vi "MassData Parameter Support Demo.vi"() -> ()   [LabVIEW 2017]
uses:
  addons/MassData-Parameter/Utility/Def-MassData Status Indicator(Vertical).ctl
  e399a5d2-a107-417c-bf24-9f3d5e5cdf18.vi
  6831a10e-81b1-43f0-9df7-fec7c9a78c49.vi
  49f32103-30ee-4ef6-a51c-53b3f34b46c3.vi
  addons/MassData-Parameter/_support/FGV-MassData(lvlibp).vi
  <userlib>/_NEVSTOP/Communicable State Machine(CSM)/Utility/CSM Data Type String.vi
  addons/MassData-Parameter/CSM MassData Parameter Support.lvlib
panel:
  in  "Boolean":bool
  in  "stop":bool
  out "MassData Status":T1={"w"={287840.0, 276144.0}, "r"={287840.0, 276144.0}} {"r" scale=1.0..50000000.0 scale format="%#_6p"; "w" scale=1.0..50000000.0 scale format="%#_6p"}
  out "Argument":string
  out "Waveform Graph":i32[](graph)
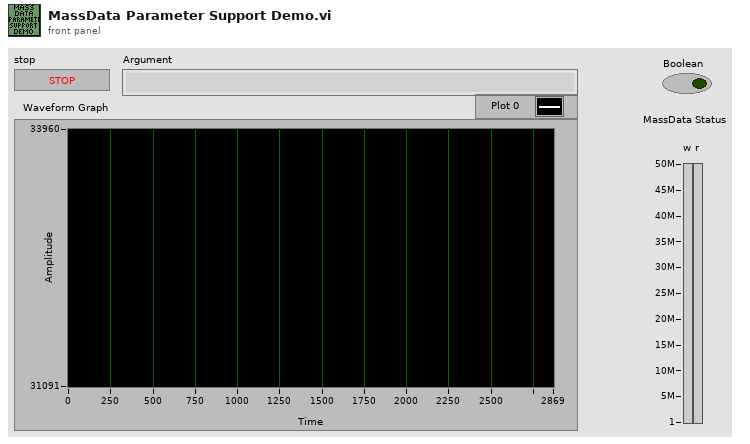
[diagram p1: front panel]
types:
  T1 = typedef "Def-MassData Status Indicator(Vertical).ctl" = cluster{"w":cluster{dbl, dbl}, "r":cluster{dbl, dbl}}
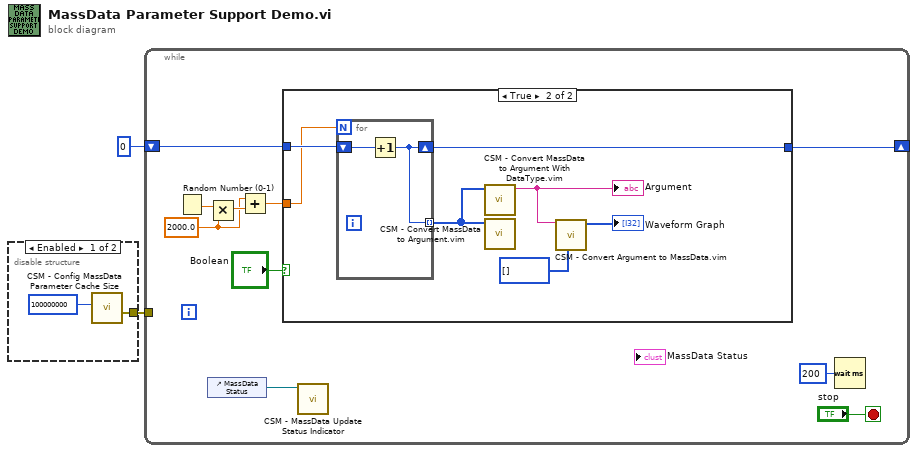
[diagram p0: block diagram]
diagram:
  n1 = disable-structure shown="Enabled" {
    disable-tunnel: [w3 _] -> w1
    frame Enabled {
      n2 = call "CSM - Config MassData Parameter Cache Size.vi"("Size (50M)"=100000000 ("size(1M)")) -> ("Error out"=w3:errorcluster)  [unwired: 10 in]
    }
    frame Disabled {
    }
  }
  n3 = while {
    shift-right: [w11] -> _
    shift-left: 0 -> [w12]
    tunnel: w1 -> [_]
    stop <- "stop" stop-if-true
    w8 = 2000.0 ("y")
    n4 = Random Number (0-1)() -> (number: 0 to 1=w10:dbl)
    n5 = Multiply(x=w10, y=w8) -> (x*y=w9:dbl)
    n6 = control-ref of="MassData Status"() -> (w6:refnum<vi>)
    n7 = Add(x=w8, y=w9) -> (x+y=w7:dbl)
    n8 = case shown="True" "Boolean" {
      tunnel: w12 -> [w15 w22]
      tunnel: [w15 w21] -> w11
      tunnel: w7 -> [_ w20]
      frame False {
      }
      frame True {
        n9 = for {
          N: w20 -> [_]
          tunnel: [w23] -> w17 mode=indexing
          shift-right: [w23] -> w21
          shift-left: w22 -> [w24]
          n10 = Increment(x=w24) -> (x+1=w23:i32)
        }
        n11 = call "CSM - Convert MassData to Argument With DataType.vim"("Data"=w17) -> ("MassData Argument"=w16:string)  [unwired: 7 in, 1 out]
        "Argument" <- w16
        n12 = call "CSM - Convert MassData to Argument.vim"("Data"=w17) -> ()  [unwired: 7 in, 2 out]
        n13 = call "CSM - Convert Argument to MassData.vim"("Type"=i32[] [], "MassData Argument"=w16) -> ("Data"=→"Waveform Graph":i32[])  [unwired: 6 in, 1 out]
      }
    }
    n14 = call "CSM - MassData Update Status Indicator.vi"("MassData Status Indicator"=w6) -> ()  [unwired: 10 in, 1 out]
    n15 = Wait (ms)(milliseconds to wait=u32 200) -> ()  [unwired: 1 out]
  }
